vi "Address Publish Message.vi"(9 "Return Priority (Normal)":T1=enum."Normal", 10 "Mediator Enqueuer":refnum<class "Message Enqueuer.lvclass">, 11 "Publish Msg in":refnum<class "Publish Msg.lvclass">) -> (3 "Publish Msg out":refnum<class "Publish Msg.lvclass">)   [LabVIEW 2020, in "IMediator.lvlib" / "Publish Msg.lvclass"]
uses:
  Publish Msg.lvclass
  <vilib>/ActorFramework/Message Enqueuer/Message Enqueuer.lvclass
  <vilib>/ActorFramework/Message Enqueuer/Message Priority.ctl
  composed-af-messages/Source/RoundTripMessage/RoundTripMessage.lvclass/RoundTripMessage.ctl
  composed-af-messages/Source/RoundTripMessage/RoundTripMessage.lvclass
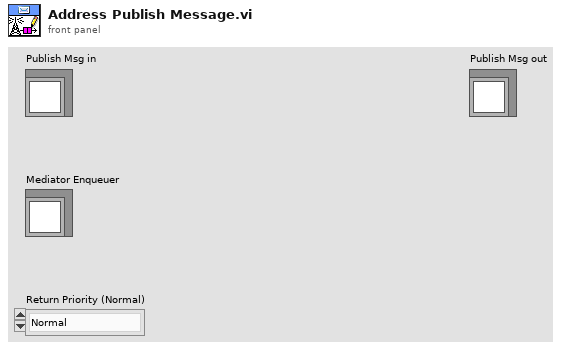
[diagram p1: front panel]
types:
  T1 = typedef "Actor Framework.lvlib/Message Enqueuer.lvclass/Message Priority.ctl" = enum16{"Low", "Normal", "High"}
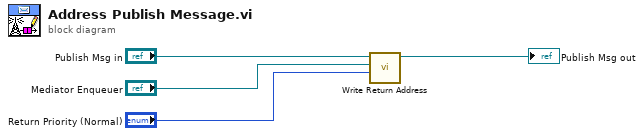
[diagram p0: block diagram]
diagram:
  n1 = call "Write Return Address.vi"("Return Priority (Normal)"="Return Priority (Normal)", "Return Enqueuer"="Mediator Enqueuer", "RoundTripMessage In"="Publish Msg in") -> ("RoundTripMessage Out"=→"Publish Msg out":refnum<class "Publish Msg.lvclass">)  [unwired: 8 in]
